vi "DllFxpSinAndCosTemp.vi"(6 "ready for output":bool, 8 "input valid":bool, 11 "phase":fxp<+/-,64,32>) -> (0 "output valid":bool, 2 "cos":fxp<+,1,1>, 3 "sin":fxp<+,1,1>, 4 "ready for input":bool)   [LabVIEW 2017]
uses:
  <vilib>/rvi/FXPMathLib/FxpSinAndCos/subVIs/nifxpmath_SinAndCos_SimConfig.ctl
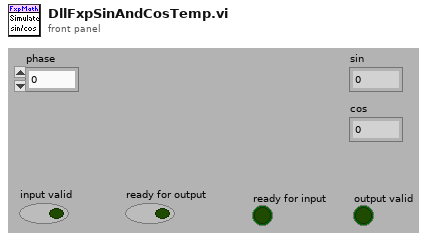
[diagram p1: front panel]
types:
  T1 = typedef "nifxpmath_SinAndCos_SimConfig.ctl" = cluster{"kPhaseLen":u16, "kPhaseIwl":i16, "kPhaseSigned":bool, "kSinCosLen":u16, "kInputRegister":bool, "kOutputRegister":bool, "kCoarseRotation":bool, "kPrecision":u16, "kIteration":u16, "QuantiMode":u16, "HandShake":bool, "CycleLimit":u16, "StrictLimit":bool}
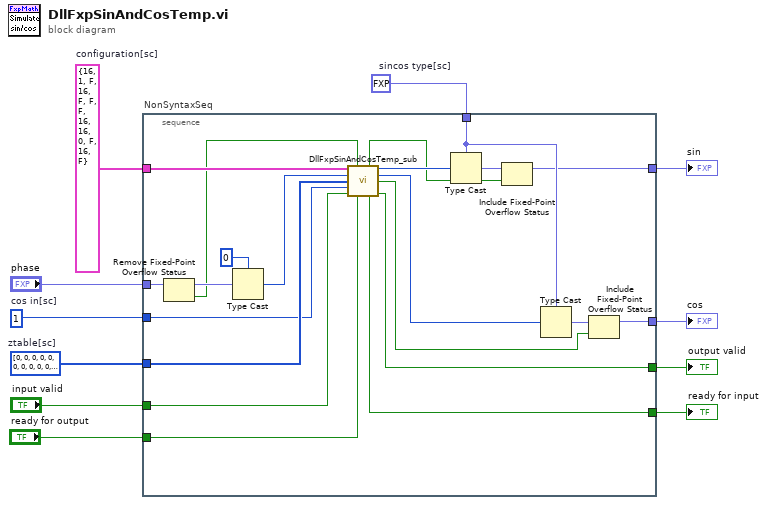
[diagram p0: block diagram]
diagram:
  w1 = T1 {"kPhaseLen"=16, "kPhaseIwl"=1, "kPhaseSigned"=FALSE, "kSinCosLen"=16, "kInputRegister"=FALSE, "kOutputRegister"=FALSE, "kCoarseRotation"=FALSE, "kPrecision"=16, "kIteration"=16, "QuantiMode"=0, "HandShake"=FALSE, "CycleLimit"=16, "StrictLimit"=FALSE}  # configuration[sc]
  w3 = u64[] [0, 0, 0, 0, 0, 0, 0, 0, 0, 0, 0, 0, 0, 0, 0, 0]  # ztable[sc]
  w7 = u64 1  # cos in[sc]
  w6 = fxp<+,1,1> 0.0  # sincos type[sc]
  n1 = stacked-sequence "NonSyntaxSeq" {
    tunnel: "phase" -> [w32]
    tunnel: "input valid" -> [w19]
    tunnel: [w27] -> w5
    tunnel: [w26] -> w4
    tunnel: [w13] -> w10
    tunnel: [w12] -> w9
    tunnel: w1 -> [w24]
    tunnel: w7 -> [w20]
    tunnel: w3 -> [w21]
    tunnel: w6 -> [w30]
    tunnel: "ready for output" -> [w18]
    frame #0 {
      n2 = Remove Fixed-Point Overflow Status(3:w32) -> (0:w22:bool, 1:w28:fxp<+/-,64,32>)
      n3 = Type Cast(type=u64 0, x=w28) -> (*(type *) &x=w23:u64)
      n4 = call <vilib>:"DllFxpSinAndCosTemp_sub.vi"("configuration[sc]"=w24, "phase ovfl status"=w22, "phase"=w23, "ztable"=w21, "cos initial"=w20, "input valid"=w19, "ready for output"=w18) -> ("sin ovfl status"=w16:bool, "sin"=w17:u64, "cos"=w15:u64, "cos ovfl status"=w14:bool, "ready for input"=w12:bool, "output valid"=w13:bool)  [unwired: 3 out]
      n5 = Type Cast(type=w30, x=w17) -> (*(type *) &x=w29:fxp<+,1,1>)
      n6 = Include Fixed-Point Overflow Status(2:w16, 3:w29) -> (1:w27:fxp<+,1,1>)
      n7 = Type Cast(type=w30, x=w15) -> (*(type *) &x=w25:fxp<+,1,1>)
      n8 = Include Fixed-Point Overflow Status(2:w14, 3:w25) -> (1:w26:fxp<+,1,1>)
    }
  }
  "output valid" <- w10
  "ready for input" <- w9
  "sin" <- w5
  "cos" <- w4
